vi "HFRR ADV v09.vi"() -> ()   [LabVIEW 2025] (continued)
                }
                n3148 = local read "TITTLE"() -> (w4088:string)
                n3149 = call-dynamic "Set Report Header Text.vi"("report in"=w4071, "center header text"=w4088, "error in (no error)"=w4070) -> ("report out"=w4109:refnum<class "NI_report.lvclass">, "error out"=w4108:errorcluster)  [unwired: 11 in]
                n3150 = for {
                  N: 1 -> [_]
                  tunnel: [w4147] -> w4095
                  tunnel: [w4146] -> w4094
                  tunnel: w4109 -> [w4145]
                  tunnel: w4108 -> [w4144]
                  n3151 = call-dynamic "New Report Line.vi"("report in"=w4145, "error in (no error)"=w4144) -> ("report out"=w4147:refnum<class "NI_report.lvclass">, "error out"=w4146:errorcluster)  [unwired: 12 in]
                }
                n3152 = for {
                  N: 2 -> [_]
                  tunnel: [w4139] -> w4101
                  tunnel: [w4138] -> w4100
                  tunnel: w4095 -> [w4137]
                  tunnel: w4094 -> [w4136]
                  n3153 = call-dynamic "New Report Line.vi"("report in"=w4137, "error in (no error)"=w4136) -> ("report out"=w4139:refnum<class "NI_report.lvclass">, "error out"=w4138:errorcluster)  [unwired: 12 in]
                }
                n3154 = for {
                  N: 25 -> [_]
                  tunnel: w4101 -> [w4135]
                  tunnel: w4100 -> [w4133]
                  tunnel: [w4134] -> w4104
                  tunnel: [w4132] -> w4103
                  n3155 = call-dynamic "Set Report Tab Width.vi"("report in"=w4135, "error in (no error)"=w4133) -> ("report out"=w4134:refnum<class "NI_report.lvclass">, "error out"=w4132:errorcluster)  [unwired: 12 in]
                }
                n3156 = control-ref of="Tab Control 9"() -> (w4099:refnum<vi>)
                n3157 = call-dynamic "Append Control Image to Report.vi"("report in"=w4104, "alignment (default)"=HTML_Report_Image_Alignment."ABSMIDDLE", "ctrl reference"=w4099, "error in (no error)"=w4103) -> ("report out"=w4098:refnum<class "NI_report.lvclass">, "error out"=w4097:errorcluster)  [unwired: 8 in, 2 out]
                n3158 = for {
                  N: 3 -> [_]
                  tunnel: [w4131] -> w4082
                  tunnel: [w4130] -> w4081
                  tunnel: w4098 -> [w4129]
                  tunnel: w4097 -> [w4128]
                  n3159 = call-dynamic "New Report Line.vi"("report in"=w4129, "error in (no error)"=w4128) -> ("report out"=w4131:refnum<class "NI_report.lvclass">, "error out"=w4130:errorcluster)  [unwired: 12 in]
                }
                n3160 = for {
                  N: 100 -> [_]
                  tunnel: w4082 -> [w4127]
                  tunnel: w4081 -> [w4125]
                  tunnel: [w4126] -> w4078
                  tunnel: [w4124] -> w4076
                  n3161 = call-dynamic "Set Report Tab Width.vi"("report in"=w4127, "error in (no error)"=w4125) -> ("report out"=w4126:refnum<class "NI_report.lvclass">, "error out"=w4124:errorcluster)  [unwired: 12 in]
                }
                n3162 = String To Path(string="C:\\LAB-IQ\\im\\Temp_resized.jpg") -> (path=w4068:path)
                n3163 = call-poly <vilib>:"Append Image to Report.vi"("report in"=w4078, "path or URL of image"=w4068, "error in (no error)"=w4076) -> ("report out"=w4077:refnum<class "NI_report.lvclass">, "error out"=w4075:errorcluster)  [unwired: 9 in, 2 out]
                n3164 = call-poly <vilib>:"Open HTML Report in Browser.vi"("report in"=w4077, "error in (no error)"=w4075) -> ("report out"=w4112:refnum<class "NI_report.lvclass">, "error out"=w4111:errorcluster)  [unwired: 11 in, 1 out]
                n3165 = call-dynamic "Dispose Report.vi"("report in"=w4112, "error in (no error)"=w4111) -> ()  [unwired: 13 in, 1 out]
              }
              frame #2 {
              }
              frame #3 {
                n3166 = disable-structure shown="Disabled" {
                  frame Disabled {
                    n3167 = local read "String 10"() -> (w4152:string)
                    n3168 = Concatenate Strings("C:\\LAB-IQ-NXT\\Data\\" ("string"), w4152, ".jpg" ("string")) -> (w4150:string)
                    n3169 = String To Path(string=w4150) -> (path=w4149:path)
                    n3170 = Delete(path (use dialog)=w4149) -> ()  [unwired: 4 in, 3 out]
                  }
                  frame Enabled {
                  }
                }
                n3171 = local write "Print 2"(FALSE ("Print")) -> ()
              }
            }
          }
        }
      }
    }
    n3172 = property on="SetTemp" class="DigNum (strict)"("Disabled"=w2040) -> ()  [unwired: 2 in, 2 out]
    n3173 = Multiply(x=w2029, y=w2031) -> (x*y=w2030:dbl)
    n3174 = local read "MWSD"() -> (w2028:dbl)
    n3175 = Add(x=w2030, y=w2028) -> (x+y=→"WS1.4":dbl)
    n3176 = Wait (ms)(milliseconds to wait=u32 50) -> ()  [unwired: 1 out]
    n3177 = Wait (ms)(milliseconds to wait=u32 50) -> ()  [unwired: 1 out]
    n3178 = local read "Quit"() -> (w2027:bool)
  }
  n3179 = VISA Close(VISA resource name=w48, error in (no error)=w47) -> (error out=w45:errorcluster)
  n3180 = VISA Close(VISA resource name=w29, error in (no error)=w28) -> ()  [unwired: 1 out]
  n3181 = call <vilib>:"Clear Errors.vi"("error in (no error)"=w45) -> ()  [unwired: 5 in, 2 out]
  n3182 = Or(x=w35, y=w34) -> (x .or. y?=w36:bool)
  n3183 = while {
    tunnel: [w4300] -> w41
    shift-right: [w4338] -> _
    shift-left: "" -> [w4326]
    tunnel: [w4314] -> _
    i -> [w4314]
    stop <- w4300 stop-if-true
    w4340 = ";" ("string")
    n3184 = local read "start en"() -> (w4359:bool)
    n3185 = And(x="st enable", y=w4359) -> (x .and. y?=w4360:bool)
    n3186 = local read "ACQUIRE 3"() -> (w4303:bool)
    n3187 = local read "Elapsed time"() -> (w4322:dbl)
    n3188 = case shown="True" w4360 {
      tunnel: "st enable" -> [w4424 w4425]
      tunnel: [w4424 w4425] -> w4304
      frame False {
      }
      frame True {
        n3189 = local write "start en"(FALSE ("start en")) -> ()
      }
    }
    n3190 = Wait (ms)(milliseconds to wait=u32 80) -> ()  [unwired: 1 out]
    n3191 = local read "Stroke"() -> (w4313:dbl)
    n3192 = Greater?(x=w4322, y=0.1) -> (0:w4320:bool)
    n3193 = Or(x=w4304, y=w4303) -> (x .or. y?=w4305:bool)
    n3194 = case shown="True" "ACQUIRE 2" {
      frame False {
      }
      frame True {
        n3195 = call "Elapsed Time13"() -> ("Time has Elapsed"=w4367:bool)  [unwired: 12 in, 7 out]
        n3196 = case shown="True" w4367 {
          frame False {
          }
          frame True {
            n3197 = local write "ACQUIRE 2"(FALSE ("ACQUIRE 2")) -> ()
            n3198 = local write "ACQUIRE 3"(FALSE ("ACQUIRE 2")) -> ()
          }
        }
        n3199 = local write "ACQUIRE 3"(TRUE ("ACQUIRE 2")) -> ()
      }
    }
    n3200 = case shown="True" w4305 {
      tunnel: w4313 -> [_ w4447]
      tunnel: [w4427 _] -> w4357
      tunnel: w4320 -> [_ _]
      tunnel: w4303 -> [_ w4434]
      frame False {
        w4427 = TRUE ("PID Rst")
        n3201 = local read "stop cmd"() -> (w4428:bool)
        n3202 = case shown="True" w4428 {
          frame False {
          }
          frame True {
            n3203 = local write "stop cmd"(FALSE ("stop cmd")) -> ()
          }
        }
        n3204 = local write "PID Rst"(TRUE ("PID Rst")) -> ()
        "start en" <- w4427
      }
      frame True {
        w4454 = cluster{"output high":dbl, "output low":dbl} {"output high"=600.0, "output low"=-600.0} ("output range")
        n3205 = local read "STROKE GAIN :"() -> (w4439:dbl)
        n3206 = call "Elapsed Time6"("Reset"="PID Rst", "Auto Reset"=FALSE) -> ("Time has Elapsed"=w4448:bool)  [unwired: 10 in, 7 out]
        n3207 = Multiply(x="Set Strk", y=w4439) -> (x*y=w4432:dbl)
        n3208 = case shown="False" w4448 {
          tunnel: [w4459 w4460] -> w4451
          tunnel: "Set Strk" -> [w4459 _]
          tunnel: w4447 -> [_ w4460]
          frame False {
          }
          frame True {
          }
        }
        n3209 = Multiply(x=w4432, y=1.0) -> (x*y=w4431:dbl)
        n3210 = Select(t=T8 {"Proportional Gain (Kc)"=0.0, "Integral Time (Ti, min)"=0.02, "Derivative Time (Td, min)"=0.0} ("Stroke PID Gains"), s=w4434, f="Stroke PID Gains") -> (s? t:f=w4435:T8)
        n3211 = Not(x=w4448) -> (.not. x?=w4446:bool)
        n3212 = call-poly <vilib>:"PID.vi"("reinitialize? (F)"=w4446, "output range"=w4454, "PID gains"=w4435, "process variable"=w4451, "setpoint"="Set Strk") -> ("output"=w4445:dbl)  [unwired: 5 in, 1 out]
        "Stroke PID OUT" <- w4445
        n3213 = Select(t=w4445, s=w4448, f=0.0) -> (s? t:f=w4449:dbl)
        n3214 = flat-sequence {
          tunnel: w4449 -> [_]
          frame #0 {
            n3215 = local write "PID Rst"(FALSE ("PID Rst")) -> ()
          }
        }
        n3216 = Add(x=w4431, y=w4449) -> (x+y=w4444:dbl)
        n3217 = Unbundle(w4454) -> ("output high"=w4453:dbl, "output low"=w4452:dbl)
        n3218 = To Word Integer(number=w4444) -> (16bit integer=w4441:i16)
        n3219 = property on="Stroke PID OUT" class="Slide (strict)"("Scale.Range:Minimum"=w4452, "Scale.Range:Maximum"=w4453) -> ()  [unwired: 2 in, 2 out]
        n3220 = In Range and Coerce(upper limit=4095.0 ("f"), x=w4441, lower limit=100.0 ("f")) -> (coerced(x)=w4438:dbl)  [unwired: 1 out]
        "PID Out" <- w4438
        n3221 = Number To Decimal String(number=w4438) -> (decimal integer string=→"st gain":string)  [unwired: 1 in]
        "stop cmd" <- TRUE ("Auto Reset")
      }
    }
    n3222 = flat-sequence {
      frame #0 {
        n3223 = local read "CH-POWER +"() -> (w4371:u16)
        n3224 = local read "CH-POWER -"() -> (w4372:u16)
        n3225 = case shown="1" w4372 {
          tunnel: "PWR" -> [w4373 w4374 w4375 w4376 w4377 w4378 w4379 w4380]
          frame 0, Default {
            n3226 = local write "Do 0"(w4373) -> ()
          }
          frame 1 {
            n3227 = local write "Do 1"(w4374) -> ()
          }
          frame 2 {
            n3228 = local write "Do 2"(w4375) -> ()
          }
          frame 3 {
            n3229 = local write "Do 3"(w4376) -> ()
          }
          frame 4 {
            n3230 = local write "Do 4"(w4377) -> ()
          }
          frame 5 {
            n3231 = local write "Do 5"(w4378) -> ()
          }
          frame 6 {
            n3232 = local write "Do 6"(w4379) -> ()
          }
          frame 7 {
            n3233 = local write "Do 7"(w4380) -> ()
          }
        }
        n3234 = case shown="1" w4371 {
          tunnel: "PWR" -> [w4381 w4382 w4383 w4384 w4385 w4386 w4387 w4388]
          frame 0, Default {
            n3235 = local write "Do 0"(w4381) -> ()
          }
          frame 1 {
            n3236 = local write "Do 1"(w4382) -> ()
          }
          frame 2 {
            n3237 = local write "Do 2"(w4383) -> ()
          }
          frame 3 {
            n3238 = local write "Do 3"(w4384) -> ()
          }
          frame 4 {
            n3239 = local write "Do 4"(w4385) -> ()
          }
          frame 5 {
            n3240 = local write "Do 5"(w4386) -> ()
          }
          frame 6 {
            n3241 = local write "Do 6"(w4387) -> ()
          }
          frame 7 {
            n3242 = local write "Do 7"(w4388) -> ()
          }
        }
      }
    }
    n3243 = local read "RUN"() -> (w4311:bool)
    n3244 = Or(x=w4311, y="ACQUIRE 3") -> (x .or. y?=w4310:bool)
    n3245 = local read "Set Hz"() -> (w4328:dbl)
    n3246 = Select(t=w4328, s=w4310, f=0.0) -> (s? t:f=w4327:dbl)
    n3247 = local read "st gain"() -> (w4331:string)
    n3248 = local read "DO"() -> (w4332:string)
    n3249 = case shown="True" "Boolean 10" {
      frame False {
      }
      frame True {
        n3250 = local write "Tab Control 8"(enum32{"setup", "calibrate"}."calibrate" ("Tab Control 8")) -> ()
        n3251 = local write "Boolean 10"(FALSE ("Boolean 10")) -> ()
      }
    }
    n3252 = Number To Decimal String(number=w4327) -> (decimal integer string=w4330:string)  [unwired: 1 in]
    n3253 = case shown="True" "Boolean 11" {
      frame False {
      }
      frame True {
        n3254 = local write "Tab Control 8"(enum32{"setup", "calibrate"}."setup" ("Tab Control 8")) -> ()
        n3255 = local write "Boolean 11"(FALSE ("Boolean 11")) -> ()
      }
    }
    n3256 = String Length(string=w4331) -> (length=w4346:i32)
    n3257 = String Length(string=w4332) -> (length=w4334:i32)
    n3258 = String Length(string=w4330) -> (length=w4347:i32)
    n3259 = Subtract(x=4.0, y=w4346) -> (x-y=w4343:dbl)
    n3260 = Subtract(x=3.0, y=w4334) -> (x-y=w4337:dbl)
    n3261 = flat-sequence {
      tunnel: w4357 -> [_]
      frame #0 {
        n3262 = Build Array("Do 0", "Do 1", "Do 2", "Do 3", "Do 4", "Do 5", "Do 6", "Do 7") -> (w4415:bool[])
        n3263 = Boolean Array To Number(Boolean array=w4415) -> (number=w4413:u32)
        n3264 = Add(x=w4413, y=u32 0) -> (x+y=w4411:u32)
        n3265 = Number To Decimal String(number=w4411) -> (decimal integer string=→"DO":string)  [unwired: 1 in]
      }
    }
    n3266 = Subtract(x=3.0, y=w4347) -> (x-y=w4348:dbl)
    n3267 = Replace Substring(3:w4343, 4:w4331, 5:"0000" ("string")) -> (1:w4341:string)  [unwired: 1 in, 1 out]
    n3268 = Replace Substring(3:w4337, 4:w4332, 5:"000" ("string")) -> (1:w4333:string)  [unwired: 1 in, 1 out]
    n3269 = Replace Substring(3:w4348, 4:w4330, 5:"000" ("string")) -> (1:w4342:string)  [unwired: 1 in, 1 out]
    n3270 = Concatenate Strings("*" ("string"), w4342, w4340, w4341, w4340, w4333, "$" ("string")) -> (w4338:string)
    "Stroke_send_Val" <- w4338
    n3271 = local read "RUN"() -> (w4308:bool)
    n3272 = local read "ACQUIRE 3"() -> (w4307:bool)
    n3273 = local read "send"() -> (w4324:bool)
    n3274 = Not Equal?(x=w4326, y=w4338) -> (x != y?=w4339:bool)
    n3275 = Or(x=w4308, y=w4307) -> (x .or. y?=w4306:bool)
    n3276 = And(x=w4324, y=w4306) -> (x .and. y?=w4323:bool)
    n3277 = Or(x=w4339, y=w4323) -> (x .or. y?=w4317:bool)
    n3278 = case shown="False" w4306 {
      frame False {
        "send" <- TRUE ("send")
      }
      frame True {
      }
    }
    n3279 = call "Elapsed Time4"("Time Target (s)"=0.5) -> ("Time has Elapsed"=w4315:bool)  [unwired: 11 in, 7 out]
    n3280 = local read "Din"() -> (w4356:u8[])
    n3281 = Or(x=w4315, y=w4317) -> (x .or. y?=w4316:bool)
    n3282 = local read "Quit"() -> (w4300:bool)
    n3283 = Index Array(array=w4356, index=0) -> (element=w4354:u8)
    n3284 = case shown="True" w4316 {
      tunnel: w4338 -> [_ w4392]
      frame False {
      }
      frame True {
        n3285 = local read "Due Com"() -> (w4393:string[])
        n3286 = Build Array (concatenate)(w4393, w4392) -> (→"Due Com":string[])
        n3287 = local write "send"(FALSE ("send")) -> ()
      }
    }
    n3288 = Number To Boolean Array(number=w4354) -> (Boolean array=w4353:bool[])
    n3289 = Array Size(array=w4353) -> (size(s)=w4352:i32)
    n3290 = Greater Than 0?(x=w4352) -> (x > 0?=w4351:bool)
    n3291 = case shown="True" w4351 {
      tunnel: w4353 -> [_ w4407]
      frame False {
      }
      frame True {
        n3292 = Index Array(array=w4407, index #1=0 ("index"), index #2=1 ("index"), index #3=2 ("index"), index #4=3 ("index"), index #5=4 ("index"), index #6=5 ("index"), index #7=6 ("index"), index #8=7 ("index")) -> (element #1=→"DI 0":bool, element #2=→"DI 1":bool, element #3=→"DI 2":bool, element #4=→"DI 3":bool, element #5=→"DI 4":bool, element #6=→"DI 5":bool, element #7=→"DI 6":bool, element #8=→"DI 7":bool)
      }
    }
  }
  n3293 = Or(x=w31, y=w36) -> (x .or. y?=w43:bool)
  n3294 = control-ref of="new picture"() -> ()  [unwired: 1 out]
  n3295 = Or(x=w50, y=w43) -> (x .or. y?=w40:bool)
  n3296 = Or(x=w40, y=w41) -> (x .or. y?=w32:bool)
  n3297 = while {
    tunnel: [w4462] -> w54
    tunnel: [w4463] -> _
    i -> [w4463]
    stop <- w4462 stop-if-true
    n3298 = local read "PID-out"() -> (w4464:dbl)
    "Horizontal Slider Control" <- w4464
    n3299 = Greater Or Equal?(x=w4464, y=2.0) -> (x >= y?=w4465:bool)
    n3300 = flat-sequence {
      tunnel: w4465 -> [w4473]
      tunnel: w4464 -> [w4476]
      tunnel: [w4474] -> w4471
      tunnel: [w4472] -> w4470
      tunnel: [w4492] -> w4469
      tunnel: w4471 -> [w4492]
      tunnel: w4470 -> [w4489]
      tunnel: [w4489] -> w4468
      tunnel: w4469 -> [w4494]
      tunnel: [w4493] -> w4467
      tunnel: w4468 -> [w4493]
      tunnel: w4467 -> [w4508]
      frame #0 {
        n3301 = case shown="True" w4473 {
          selector: w4473 -> [w4478 _]
          frame False {
            n3302 = local write "HEATER"(w4478) -> ()
          }
          frame True {
            w4480 = TRUE ("data")
            n3303 = local read "CH-HEATER"() -> (w4479:u16)
            n3304 = case shown="2" w4479 {
              tunnel: w4480 -> [w4481 w4482 w4483 w4484 w4485 w4486 w4487 w4488]
              frame 0, Default {
                n3305 = local write "Do 0"(w4481) -> ()
              }
              frame 1 {
                n3306 = local write "Do 1"(w4482) -> ()
              }
              frame 2 {
                n3307 = local write "Do 2"(w4483) -> ()
              }
              frame 3 {
                n3308 = local write "Do 3"(w4484) -> ()
              }
              frame 4 {
                n3309 = local write "Do 4"(w4485) -> ()
              }
              frame 5 {
                n3310 = local write "Do 5"(w4486) -> ()
              }
              frame 6 {
                n3311 = local write "Do 6"(w4487) -> ()
              }
              frame 7 {
                n3312 = local write "Do 7"(w4488) -> ()
              }
            }
            "HEATER" <- w4480
          }
        }
        n3313 = Select(t=w4476, s=w4473, f=0.0) -> (s? t:f=w4472:dbl)
        n3314 = Greater Or Equal?(x=w4476, y=97.0) -> (x >= y?=w4474:bool)
      }
      frame #1 {
        n3315 = Multiply(x=w4489, y=5.0) -> (x*y=w4491:dbl)
        n3316 = Wait (ms)(milliseconds to wait=w4491) -> ()  [unwired: 1 out]
      }
      frame #2 {
        n3317 = case shown="False" w4494 {
          frame False {
            w4495 = FALSE ("data")
            n3318 = local read "CH-HEATER"() -> (w4496:u16)
            n3319 = case shown="4" w4496 {
              tunnel: w4495 -> [w4497 w4498 w4499 w4500 w4501 w4502 w4503 w4504]
              frame 0, Default {
                n3320 = local write "Do 0"(w4497) -> ()
              }
              frame 1 {
                n3321 = local write "Do 1"(w4498) -> ()
              }
              frame 2 {
                n3322 = local write "Do 2"(w4499) -> ()
              }
              frame 3 {
                n3323 = local write "Do 3"(w4500) -> ()
              }
              frame 4 {
                n3324 = local write "Do 4"(w4501) -> ()
              }
              frame 5 {
                n3325 = local write "Do 5"(w4502) -> ()
              }
              frame 6 {
                n3326 = local write "Do 6"(w4503) -> ()
              }
              frame 7 {
                n3327 = local write "Do 7"(w4504) -> ()
              }
            }
            n3328 = local write "HEATER"(w4495) -> ()
          }
          frame True {
          }
        }
      }
      frame #3 {
        n3329 = Subtract(x=100, y=w4508) -> (x-y=w4507:dbl)
        n3330 = Multiply(x=w4507, y=5.0) -> (x*y=w4505:dbl)
        n3331 = Wait (ms)(milliseconds to wait=w4505) -> ()  [unwired: 1 out]
      }
    }
    n3332 = local read "Quit"() -> (w4462:bool)
  }
  n3333 = Or(x=w54, y=w32) -> (x .or. y?=w53:bool)
  n3334 = while {
    tunnel: [w4510] -> w49
    i -> [w4517]
    stop <- w4510 stop-if-true
    n3335 = local read "Quit"() -> (w4510:bool)
    n3336 = Equal To 0?(x=w4517) -> (x = 0?=w4515:bool)
    n3337 = call "Elapsed Time3"("Time Target (s)"=45.0, "Auto Reset"=TRUE) -> ("Time has Elapsed"=w4514:bool)  [unwired: 10 in, 7 out]
    n3338 = Wait (ms)(milliseconds to wait=u32 50) -> ()  [unwired: 1 out]
    n3339 = Or(x=w4514, y=w4515) -> (x .or. y?=w4516:bool)
    n3340 = case shown="True" w4516 {
      frame False {
      }
      frame True {
        n3341 = call <vilib>:"System Exec.vi"("run minimized? (F)"=TRUE, "error in (no error)"="error in (no error)", "command line"="powercfg.exe -change -monitor-timeout-ac 0") -> ("error out"=w4528:errorcluster)  [unwired: 5 in, 3 out]
        n3342 = call <vilib>:"System Exec.vi"("run minimized? (F)"=TRUE, "error in (no error)"=w4528, "command line"="powercfg.exe -change -disk-timeout-ac 0") -> ("error out"=w4527:errorcluster)  [unwired: 5 in, 3 out]
        n3343 = call <vilib>:"System Exec.vi"("run minimized? (F)"=TRUE, "error in (no error)"=w4527, "command line"="powercfg.exe -change -standby-timeout-ac 0") -> ("error out"=w4526:errorcluster)  [unwired: 5 in, 3 out]
        n3344 = call <vilib>:"System Exec.vi"("run minimized? (F)"=TRUE, "error in (no error)"=w4526, "command line"="powercfg.exe -change -hibernate-timeout-ac 0") -> ("error out"=w4525:errorcluster)  [unwired: 5 in, 3 out]
        n3345 = call <vilib>:"Simple Error Handler.vi"("error in (no error)"=w4525) -> ("error out"=w4531:errorcluster)  [unwired: 4 in, 4 out]
        n3346 = call <vilib>:"Clear Errors.vi"("error in (no error)"=w4531) -> ("error out"=→"error out":errorcluster)  [unwired: 5 in, 1 out]
      }
    }
  }
  n3347 = Compound Arithmetic op=OR(w52, w53, w49) -> (w51:bool)
  n3348 = flat-sequence {
    tunnel: w51 -> [_]
    tunnel: [w4533] -> w9
    tunnel: w9 -> [_]
    frame #0 {
      n3349 = call "CLOSE CONNECTION.vi"() -> ("error out"=w4533:errorcluster)  [unwired: 11 in]
    }
    frame #1 {
      n3350 = Quit LabVIEW(quit? (T)=TRUE) -> ()
      n3351 = local write "Quit"(FALSE ("EXIT")) -> ()
    }
  }
  n3352 = property on="Heater Button" class="Bool (strict)"("Visible"=TRUE) -> ()  [unwired: 2 in, 2 out]
  n3353 = disable-structure shown="Disabled" {
    disable-tunnel: _ -> [w4539 _]
    disable-tunnel: _ -> [w4536 _]
    disable-tunnel: _ -> [w4537 _]
    frame Disabled {
      n3354 = disable-structure shown="Disabled" {
        disable-tunnel: [w4546 _] -> w4538
        frame Disabled {
          n3355 = while {
            shift-right: [w4588] -> w4544
            shift-left: errorcluster {"status"=TRUE, "code"=0, "source"="Init"} ("error out") -> [w4553]
            shift-right: [w4587] -> w4543
            shift-left: _ -> [w4554]
            shift-right: [w4586] -> _
            shift-left: "" -> [w4585]
            tunnel: [w4547] -> w4546
            shift-right: ["Set Rh"] -> _
            shift-left: 0.0 ("Set Rh") -> [w4579]
            tunnel: [w4556] -> _
            i -> [w4556]
            stop <- w4547 stop-if-true
            n3356 = flat-sequence {
              tunnel: w4553 -> [w4591]
              tunnel: [w4591] -> w4552
              frame #0 {
                n3357 = Wait (ms)(milliseconds to wait=u32 200) -> ()  [unwired: 1 out]
              }
            }
            n3358 = local read "Com Port 3"() -> (w4555:refnum<visa-resource-name>)
            n3359 = local read "Humidity Str Rec"() -> (w4557:string)
            n3360 = Not Equal?(x="Set Rh", y=w4579) -> (x != y?=w4584:bool)
            n3361 = Number To Decimal String(number="Set Rh") -> (decimal integer string=w4582:string)  [unwired: 1 in]
            n3362 = Not Equal?(x=w4555, y=w4554) -> (x != y?=w4550:bool)
            n3363 = Concatenate Strings("#setPoint00" ("string"), w4582) -> (w4583:string)
            n3364 = case shown="False" w4584 {
              tunnel: w4583 -> [_ w4603]
              frame False {
                n3365 = local read "Humidity"() -> (w4600:bool)
                n3366 = case shown="True" w4600 {
                  frame False {
                    n3367 = local write "Humidity Str Send"("stop" ("Humidity Str Send")) -> ()
                  }
                  frame True {
                    n3368 = local write "Humidity Str Send"("start" ("Humidity Str Send")) -> ()
                  }
                }
              }
              frame True {
                n3369 = local write "Humidity Str Send"(w4603) -> ()
              }
            }
            n3370 = Or(x=w4550, y="Re-Initialise") -> (x .or. y?=w4549:bool)
            n3371 = String Subset(string=w4557, offset (0)=7) -> (substring=w4572:string)  [unwired: 1 in]
            n3372 = Match Pattern(string=w4557, regular expression="?") -> (offset past match=w4575:i32)  [unwired: 1 in, 3 out]
            n3373 = Match Pattern(string=w4557, regular expression="v") -> (offset past match=w4578:i32)  [unwired: 1 in, 3 out]
            n3374 = case shown="True" w4549 {
              tunnel: w4552 -> [w4589 _]
              tunnel: [w4589 errorcluster {"status"=TRUE, "code"=0, "source"="Init"} ("error out")] -> w4551
              frame False {
              }
              frame True {
              }
            }
            n3375 = Equal?(x=w4575, y=-1) -> (x = y?=w4559:bool)
            n3376 = Match Pattern(string=w4572, regular expression="g") -> (after substring=w4573:string, offset past match=w4564:i32)  [unwired: 1 in, 2 out]
            n3377 = Match Pattern(string=w4572, regular expression="y") -> (after substring=w4571:string, offset past match=w4565:i32)  [unwired: 1 in, 2 out]
            n3378 = Greater?(x=w4565, y=w4564) -> (0:w4570:bool)
            n3379 = Greater Or Equal To 0?(x=w4565) -> (x >= 0?=w4562:bool)
            n3380 = Greater Or Equal To 0?(x=w4564) -> (x >= 0?=w4563:bool)
            n3381 = Or(x=w4562, y=w4563) -> (x .or. y?=w4561:bool)
            n3382 = Greater Or Equal To 0?(x=w4578) -> (x >= 0?=w4560:bool)
            n3383 = Select(t=w4571, s=w4570, f=w4573) -> (s? t:f=w4566:string)
            n3384 = case shown="Error" w4551 {
              selector: w4551 -> [w4616 w4662]
              tunnel: [w4614 w4655] -> w4588
              tunnel: w4554 -> [w4617 w4661]
              tunnel: [w4615 w4664] -> w4587
              tunnel: w4585 -> [w4604 w4663]
              tunnel: [w4611 w4663] -> w4586
              frame No Error {
                n3385 = call "Elapsed Time7"() -> ("Time has Elapsed"=w4610:bool)  [unwired: 12 in, 7 out]
                n3386 = Not Equal?(x="Humidity Str Send", y=w4604) -> (x != y?=w4606:bool)
                n3387 = Or(x=w4606, y=w4610) -> (x .or. y?=w4609:bool)
                n3388 = Select(t="Humidity Str Send", s=w4606, f="vals" ("regular expression")) -> (s? t:f=w4605:string)
                n3389 = Or(x=w4609, y="Send") -> (x .or. y?=w4613:bool)
                n3390 = case shown="True" w4613 {
                  tunnel: [w4620 w4625] -> w4614
                  tunnel: w4617 -> [w4619 w4633]
                  tunnel: w4616 -> [w4620 w4632]
                  tunnel: [w4619 w4626] -> w4615
                  tunnel: w4605 -> [_ w4631]
                  tunnel: [w4618 w4622] -> w4611
                  tunnel: "Humidity Str Send" -> [_ w4623]
                  tunnel: w4606 -> [_ w4624]
                  tunnel: w4604 -> [w4618 w4621]
                  frame False {
                  }
                  frame True {
                    n3391 = flat-sequence {
                      tunnel: w4633 -> [w4641]
                      tunnel: w4632 -> [w4640]
                      tunnel: w4631 -> [w4637]
                      tunnel: [w4639] -> w4630
                      tunnel: [w4638] -> w4629
                      tunnel: w4630 -> [w4644]
                      tunnel: w4629 -> [w4643]
                      tunnel: [w4644] -> w4628
                      tunnel: [w4643] -> w4627
                      tunnel: w4628 -> [w4651]
                      tunnel: w4627 -> [w4650]
                      tunnel: [w4649] -> w4626
                      tunnel: [w4648] -> w4625
                      frame #0 {
                        n3392 = local write "Ser Led"(TRUE ("Boolean 4")) -> ()
                        n3393 = Concatenate Strings(w4637, "\r") -> (w4636:string)
                        n3394 = VISA Write(VISA resource name=w4641, write buffer=w4636, error in (no error)=w4640) -> (VISA resource name out=w4639:refnum<visa-resource-name>, error out=w4638:errorcluster)  [unwired: 1 out]
                      }
                      frame #1 {
                        n3395 = Wait (ms)(milliseconds to wait="wait") -> ()  [unwired: 1 out]
                      }
                      frame #2 {
                        w4646 = FALSE ("Send")
                        n3396 = property class="Instr"(reference=w4651, error in=w4650) -> (reference out=w4652:refnum<visa-resource-name>, error out=w4653:errorcluster, "Serial Settings:Number of Bytes at Serial Port"=w4645:u32)
                        "Humidity 2" <- w4645
                        n3397 = local write "Send"(w4646) -> ()
                        n3398 = local write "Ser Led"(w4646) -> ()
                        n3399 = VISA Read(VISA resource name=w4652, byte count=w4645, error in (no error)=w4653) -> (VISA resource name out=w4649:refnum<visa-resource-name>, read buffer=→"Humidity Str Rec":string, error out=w4648:errorcluster)  [unwired: 1 out]
                      }
                    }
                    n3400 = Select(t=w4623, s=w4624, f=w4621) -> (s? t:f=w4622:string)
                  }
                }
              }
              frame Error {
                w4669 = u16 0 items=["None"=0, "XON/XOFF"=1, "RTS/CTS"=2, "DTR/DSR"=4] ("flow control")
                w4665 = u16 0 items=["None", "Odd", "Even", "Mark", "Space"] ("parity")
                w4668 = u16 10 items=["1.0"=10, "1.5"=15, "2.0"=20] ("stop bits")
                n3401 = VISA Close(VISA resource name=w4661, error in (no error)=w4662) -> (error out=w4660:errorcluster)
                n3402 = local write "humid"("" ("humid")) -> ()
                n3403 = local write "Humidity Str Rec"("" ("Humidity Str Rec")) -> ()
                n3404 = call <vilib>:"Clear Errors.vi"("error in (no error)"=w4660) -> ("error out"=w4659:errorcluster)  [unwired: 5 in, 1 out]
                n3405 = local read "Com Port 3"() -> (w4658:refnum<visa-resource-name>)
                n3406 = call-poly "VISA Configure Serial Port"("VISA resource name"=w4658, "timeout (10sec)"=u32 1000, "termination char\n(0xA = '\\n' = LF)"=u8 10 ("termination char\n(0xA = '\\n' = LF)"), "Enable Termination\nChar (T)"=FALSE ("Enable Termination Char (T)"), "baud rate (9600)"="Humidity BaudRate", "data bits (8)"=u16 8 ("data bits"), "parity (0:none)"=w4665, "error in (no error)"=w4659, "stop bits (10: 1 bit)"=w4668, "flow control (0:none)"=w4669) -> ("VISA resource name out"=w4664:refnum<visa-resource-name>, "error out"=w4655:errorcluster)  [unwired: 4 in]
              }
            }
            n3407 = Compound Arithmetic op=AND(w4560, w4559, w4561) -> (w4558:bool)
            n3408 = case shown="True" w4558 {
              tunnel: w4557 -> [_ _]
              tunnel: w4566 -> [_ w4596]
              frame False {
              }
              frame True {
                w4594 = " " ("regular expression")
                n3409 = Match Pattern(string=w4596, regular expression=" ") -> (after substring=w4598:string)  [unwired: 1 in, 3 out]
                n3410 = Match Pattern(string=w4598, regular expression=w4594) -> (before substring=→"humid":string, after substring=w4595:string)  [unwired: 1 in, 2 out]
                n3411 = Match Pattern(string=w4595, regular expression=w4594) -> (before substring=→"temp_@Rh sensor":string)  [unwired: 1 in, 3 out]
              }
            }
            n3412 = local read "Quit"() -> (w4547:bool)
          }
          n3413 = VISA Close(VISA resource name=w4543, error in (no error)=w4544) -> (error out=w4540:errorcluster)
          n3414 = call <vilib>:"Clear Errors.vi"("error in (no error)"=w4540) -> ()  [unwired: 5 in, 2 out]
        }
        frame Enabled {
        }
      }
    }
    frame Enabled {
    }
  }
  n3415 = while {
    tunnel: [w4677] -> _
    i -> [w4677]
    stop <- w4672 stop-if-true
    # "Langauage selection"
    n3416 = property on="FF Calibration g" class="WFGraph (strict)"("Plot Area:Colors:FG Color"=u32 0) -> ()  [unwired: 2 in, 2 out]
    n3417 = Equal?(x="Lan flag", y=22.0) -> ()  [unwired: 1 out]
    n3418 = disable-structure shown="Disabled" {
      frame Disabled {
        n3419 = stacked-sequence {
          frame #0 {
            n3420 = case shown="\"Russian\"" "Language Selection" {
              tunnel: [0 1] -> w4679
              frame "English", Default {
              }
              frame "Russian" {
              }
            }
            n3421 = for {
              N: 130 -> [_]
              tunnel: "Table" -> [w4688]
              tunnel: w4679 -> [w4687]
              i -> [w4686]
              n3422 = Index Array(array=w4688, index (row)=w4686, index (col)=w4687) -> (element=w4685:string)
              n3423 = case shown="4" w4686 {
                tunnel: w4685 -> [w4689 w4690 _ w4691 w4692 w4693 w4694 w4695 w4696 w4697 w4698 w4699 w4700 w4701 w4702 w4703 w4704 w4705 w4706 w4707 w4708 w4709 w4710 w4711 w4712 w4713 w4714 w4715 w4716 _ _ w4717 w4718 w4719 w4720 w4721 w4722 w4731 w4738 w4745 w4752 w4756 w4759 w4762 w4764 w4766 w4767 w4768 w4769 w4770 w4771 w4772 w4773 w4774 w4775 w4776 w4777 w4778 w4779 w4780 w4781 w4782 w4783 w4784 w4785 w4786 w4787 w4788 w4789 w4790 w4791 w4792 w4793 w4794 w4795 w4796 w4797 w4798 w4799 w4800 w4801 w4802 w4803 w4804 w4805 w4806 w4807 w4808 w4809 w4810 w4811 w4812 w4813 w4814 w4815 w4816 w4817 w4818 w4819 w4820 w4821 w4822 w4823 w4824 w4825 _ w4826 w4827 w4828 w4829 w4830 w4831 w4832 w4833 w4834 w4835 w4836 w4837 w4838 _ w4839 w4840 w4841 w4842 w4843 w4844 _]
                frame 0 {
                  n3424 = local write "S"(w4689) -> ()
                }
                frame 1 {
                  n3425 = local write "S 2"(w4690) -> ()
                }
                frame 2 {
                }
                frame 3 {
                  n3426 = local write "S 4"(w4691) -> ()
                }
                frame 4 {
                  n3427 = property on="FILE" class="Str"("Caption.Text"=w4692) -> ()  [unwired: 2 in, 2 out]
                }
                frame 5 {
                  n3428 = property on="Fuel Discription :" class="Str"("Caption.Text"=w4693) -> ()  [unwired: 2 in, 2 out]
                }
                frame 6 {
                  n3429 = property on="Remarks :" class="Str"("Caption.Text"=w4694) -> ()  [unwired: 2 in, 2 out]
                }
                frame 7 {
                  n3430 = property on="Save & Continue" class="Bool (strict)"("Boolean Text.Text"=w4695) -> ()  [unwired: 2 in, 2 out]
                }
                frame 8 {
                }
                frame 9 {
                  n3431 = property on="Set Hz" class="DigNum (strict)"("Caption.Text"=w4697) -> ()  [unwired: 2 in, 2 out]
                }
                frame 10 {
                  "String 3" <- w4698
                }
                frame 11 {
                  n3432 = property on="NORMAL LOAD" class="DigNum (strict)"("Caption.Text"=w4699) -> ()  [unwired: 2 in, 2 out]
                }
                frame 12 {
                  "String 5" <- w4700
                }
                frame 13 {
                  n3433 = property on="Set Temp" class="DigNum (strict)"("Caption.Text"=w4701) -> ()  [unwired: 2 in, 2 out]
                }
                frame 14 {
                  n3434 = local write "S 15"(w4702) -> ()
                }
                frame 15 {
                  n3435 = property on="Set Rh" class="DigNum (strict)"("Caption.Text"=w4703) -> ()  [unwired: 2 in, 2 out]
                }
                frame 16 {
                  "String 13" <- w4704
                  "String 26" <- w4704
                }
                frame 17 {
                  n3436 = local write "S 18"(w4705) -> ()
                }
                frame 18 {
                  "String 17" <- w4706
                }
                frame 19 {
                  n3437 = property on="test time" class="DigNum (strict)"("Caption.Text"=w4707) -> ()  [unwired: 2 in, 2 out]
                }
                frame 20 {
                  "String 18" <- w4708
                  "String 22" <- w4708
                }
                frame 21 {
                  n3438 = property on="Elapsed time" class="DigNum (strict)"("Caption.Text"=w4709) -> ()  [unwired: 2 in, 2 out]
                }
                frame 22 {
                  n3439 = property on="Samplingtime 2" class="DigNum (strict)"("Caption.Text"=w4710) -> ()  [unwired: 2 in, 2 out]
                }
                frame 23 {
                  "String 21" <- w4711
                }
                frame 24 {
                  n3440 = property on="Countdown" class="DigNum (strict)"("Caption.Text"=w4712) -> ()  [unwired: 2 in, 2 out]
                }
                frame 25 {
                  n3441 = property on="Countdown 2" class="DigNum (strict)"("Caption.Text"=w4713) -> ()  [unwired: 2 in, 2 out]
                }
                frame 26 {
                  n3442 = property on="Engage" class="Bool (strict)"("Boolean Text.Text"=w4714) -> ()  [unwired: 2 in, 2 out]
                }
                frame 27 {
                  n3443 = property on="Boolean  4" class="Bool (strict)"("Boolean Text.Text"=w4715) -> ()  [unwired: 2 in, 2 out]
                }
                frame 28 {
                  n3444 = property on="Test \nStatus" class="Bool (strict)"("Boolean Text.Text"=w4716) -> ()  [unwired: 2 in, 2 out]
                }
                frame 29 {
                }
                frame 30 {
                }
                frame 31 {
                  n3445 = property on="FF Calibration g" class="WFGraph (strict)"("X Scale.Name Label.Text"=w4717) -> ()  [unwired: 2 in, 2 out]
                }
                frame 32 {
                  n3446 = property on="RSTCOF" class="Bool"("Boolean Text.Text"=w4718) -> ()  [unwired: 2 in, 2 out]
                  n3447 = property on="RST FF" class="Bool"("Boolean Text.Text"=w4718) -> ()  [unwired: 2 in, 2 out]
                  n3448 = property on="RST TEMP" class="Bool"("Boolean Text.Text"=w4718) -> ()  [unwired: 2 in, 2 out]
                  n3449 = property on="RSTV1 3" class="Bool"("Boolean Text.Text"=w4718) -> ()  [unwired: 2 in, 2 out]
                  n3450 = property on="rstv2" class="Bool"("Boolean Text.Text"=w4718) -> ()  [unwired: 2 in, 2 out]
                  n3451 = property on="RSTV1 2" class="Bool"("Boolean Text.Text"=w4718) -> ()  [unwired: 2 in, 2 out]
                  n3452 = property on="RST CP" class="Bool"("Boolean Text.Text"=w4718) -> ()  [unwired: 2 in, 2 out]
                }
                frame 33 {
                  "S 61" <- w4719
                }
                frame 34 {
                  "String 23" <- w4720
                }
                frame 35 {
                  n3453 = property on="Rh Before" class="DigNum (strict)"("Caption.Text"=w4721) -> ()  [unwired: 2 in, 2 out]
                }
                frame 36 {
                  n3454 = Match Pattern(string=w4722, regular expression=",") -> (before substring=→"bs":string, after substring=→"as":string)  [unwired: 1 in, 2 out]
                  n3455 = property on="Rh After" class="DigNum (strict)"("Caption.Text"=w4722) -> ()  [unwired: 2 in, 2 out]
                }
                frame 37 {
                  n3456 = Match Pattern(string=w4731, regular expression=",") -> (before substring=w4730:string, after substring=w4729:string)  [unwired: 1 in, 2 out]
                  "bs" <- w4730
                  "as" <- w4729
                  n3457 = Concatenate Strings(w4730, w4729) -> (w4726:string)
                  n3458 = property on="Humidity before test 2" class="DigNum (strict)"("Caption.Text"=w4726) -> ()  [unwired: 2 in, 2 out]
                  n3459 = property on="Humidity before test" class="DigNum (strict)"("Caption.Text"=w4726) -> ()  [unwired: 2 in, 2 out]
                  n3460 = Concatenate Strings(w4726, "=" ("string")) -> (w4727:string)
                  n3461 = local write "S 38"(w4727) -> ()
                }
                frame 38 {
                  n3462 = Match Pattern(string=w4738, regular expression=",") -> (before substring=w4737:string, after substring=w4736:string)  [unwired: 1 in, 2 out]
                  "bs" <- w4737
                  "as" <- w4736
                  n3463 = Concatenate Strings(w4737, w4736) -> (w4733:string)
                  n3464 = property on="Humidity after test 2" class="DigNum (strict)"("Caption.Text"=w4733) -> ()  [unwired: 2 in, 2 out]
                  n3465 = Concatenate Strings(w4733, "=" ("string")) -> (w4735:string)
                  n3466 = property on="Humidity after test" class="DigNum (strict)"("Caption.Text"=w4733) -> ()  [unwired: 2 in, 2 out]
                  n3467 = local write "S 39"(w4735) -> ()
                }
                frame 39 {
                  n3468 = Match Pattern(string=w4745, regular expression=",") -> (before substring=w4744:string, after substring=w4743:string)  [unwired: 1 in, 2 out]
                  "bs" <- w4744
                  "as" <- w4743
                  n3469 = Concatenate Strings(w4744, w4743) -> (w4740:string)
                  n3470 = property on="Temperature before test 2" class="DigNum (strict)"("Caption.Text"=w4740) -> ()  [unwired: 2 in, 2 out]
                  n3471 = property on="Temperature before test" class="DigNum (strict)"("Caption.Text"=w4740) -> ()  [unwired: 2 in, 2 out]
                  n3472 = Concatenate Strings(w4740, "=" ("string")) -> (→"String 34":string)
                }
                frame 40 {
                  n3473 = Match Pattern(string=w4752, regular expression=",") -> (before substring=w4751:string, after substring=w4750:string)  [unwired: 1 in, 2 out]
                  "bs" <- w4751
                  "as" <- w4750
                  n3474 = Concatenate Strings(w4751, w4750) -> (w4747:string)
                  n3475 = property on="Temperature after test 2" class="DigNum (strict)"("Caption.Text"=w4747) -> ()  [unwired: 2 in, 2 out]
                  n3476 = Concatenate Strings(w4747, "=" ("string")) -> (→"String 35":string)
                  n3477 = property on="Temperature after test" class="DigNum (strict)"("Caption.Text"=w4747) -> ()  [unwired: 2 in, 2 out]
                }
                frame 41 {
                  n3478 = property on="AVP" class="DigNum (strict)"("Caption.Text"=w4756) -> ()  [unwired: 2 in, 2 out]
                  n3479 = property on="AVP 2" class="DigNum (strict)"("Caption.Text"=w4756) -> ()  [unwired: 2 in, 2 out]
                  n3480 = Concatenate Strings(w4756, "=" ("string")) -> (→"String 36":string)
                }
                frame 42 {
                  n3481 = property on="MWSD" class="DigNum (strict)"("Caption.Text"=w4759) -> ()  [unwired: 2 in, 2 out]
                  n3482 = property on="MWSD 2" class="DigNum (strict)"("Caption.Text"=w4759) -> ()  [unwired: 2 in, 2 out]
                  n3483 = Concatenate Strings(w4759, "=" ("string")) -> (→"String 37":string)
                }
                frame 43 {
                  n3484 = property on="HCF 2" class="DigNum (strict)"("Caption.Text"=w4762) -> ()  [unwired: 2 in, 2 out]
                  n3485 = property on="HCF" class="DigNum (strict)"("Caption.Text"=w4762) -> ()  [unwired: 2 in, 2 out]
                  n3486 = Concatenate Strings(w4762, "=" ("string")) -> (→"String 38":string)
                }
                frame 44 {
                  n3487 = Concatenate Strings(w4764, "=" ("string")) -> (→"String 39":string)
                  n3488 = property on="WS1.4 2" class="DigNum (strict)"("Caption.Text"=w4764) -> ()  [unwired: 2 in, 2 out]
                  n3489 = property on="WS1.4" class="DigNum (strict)"("Caption.Text"=w4764) -> ()  [unwired: 2 in, 2 out]
                }
                frame 45 {
                  n3490 = property on="Save Results" class="Bool (strict)"("Boolean Text.Text"=w4766) -> ()  [unwired: 2 in, 2 out]
                }
                frame 46 {
                  n3491 = local write "S 47"(w4767) -> ()
                }
                frame 47 {
                  n3492 = local write "S 48"(w4768) -> ()
                }
                frame 48 {
                  n3493 = local write "S 49"(w4769) -> ()
                }
                frame 49 {
                  n3494 = local write "S 50"(w4770) -> ()
                }
                frame 50 {
                  n3495 = local write "S 51"(w4771) -> ()
                }
                frame 51 {
                  n3496 = local write "S 52"(w4772) -> ()
                }
                frame 52 {
                  n3497 = local write "S 53"(w4773) -> ()
                }
                frame 53 {
                  n3498 = local write "S 54"(w4774) -> ()
                }
                frame 54 {
                  n3499 = local write "S 55"(w4775) -> ()
                }
                frame 55 {
                  n3500 = local write "S 56"(w4776) -> ()
                }
                frame 56 {
                  n3501 = local write "S 57"(w4777) -> ()
                }
                frame 57 {
                  n3502 = local write "S 58"(w4778) -> ()
                }
                frame 58 {
                  n3503 = local write "S 59"(w4779) -> ()
                }
                frame 59 {
                  n3504 = local write "S 60"(w4780) -> ()
                }
                frame 60 {
                  n3505 = local write "S 62"(w4781) -> ()
                }
                frame 61 {
                  n3506 = local write "S 63"(w4782) -> ()
                }
                frame 62 {
                  n3507 = local write "S 64"(w4783) -> ()
                }
                frame 63 {
                  n3508 = local write "S 65"(w4784) -> ()
                }
                frame 64 {
                  n3509 = local write "S 66"(w4785) -> ()
                }
                frame 65 {
                  n3510 = local write "S 67"(w4786) -> ()
                }
                frame 66 {
                  n3511 = local write "S 68"(w4787) -> ()
                }
                frame 67 {
                  n3512 = local write "S 69"(w4788) -> ()
                }
                frame 68 {
                  n3513 = local write "S 70"(w4789) -> ()
                }
                frame 69 {
                  n3514 = local write "S 71"(w4790) -> ()
                }
                frame 70 {
                  n3515 = local write "S 72"(w4791) -> ()
                }
                frame 71 {
                  n3516 = local write "S 73"(w4792) -> ()
                }
                frame 72 {
                  n3517 = local write "S 74"(w4793) -> ()
                }
                frame 73 {
                  n3518 = local write "S 75"(w4794) -> ()
                }
                frame 74 {
                  n3519 = local write "S 76"(w4795) -> ()
                }
                frame 75 {
                  n3520 = local write "S 77"(w4796) -> ()
                }
                frame 76 {
                  n3521 = local write "S 78"(w4797) -> ()
                }
                frame 77 {
                  n3522 = local write "S 79"(w4798) -> ()
                }
                frame 79 {
                  n3523 = property on="Sample Temperature ( °C )" class="XYGraph (strict)"("Y Scale.Name Label.Text"=w4799) -> ()  [unwired: 2 in, 2 out]
                }
                frame 80 {
                  n3524 = local write "S 81"(w4800) -> ()
                  n3525 = property on="Humidity ( %RH )" class="XYGraph (strict)"("Y Scale.Name Label.Text"=w4800) -> ()  [unwired: 2 in, 2 out]
                }
                frame 78 {
                  n3526 = property on="Air Temperature  ( °C )" class="XYGraph (strict)"("X Scale.Name Label.Text"=w4801) -> ()  [unwired: 2 in, 2 out]
                  n3527 = property on="Humidity ( %RH )" class="XYGraph (strict)"("X Scale.Name Label.Text"=w4801) -> ()  [unwired: 2 in, 2 out]
                  n3528 = property on="Sample Temperature ( °C )" class="XYGraph (strict)"("X Scale.Name Label.Text"=w4801) -> ()  [unwired: 2 in, 2 out]
                  n3529 = property on="Coefficient Of Friction" class="XYGraph (strict)"("X Scale.Name Label.Text"=w4801) -> ()  [unwired: 2 in, 2 out]
                }
                frame 81 {
                  n3530 = property on="Air Temperature  ( °C )" class="XYGraph (strict)"("Y Scale.Name Label.Text"=w4802) -> ()  [unwired: 2 in, 2 out]
                }
                frame 82 {
                  n3531 = local write "S 84"(w4803) -> ()
                }
                frame 83 {
                  n3532 = local write "S 85"(w4804) -> ()
                }
                frame 84 {
                  n3533 = local write "S 86"(w4805) -> ()
                }
                frame 85 {
                  n3534 = local write "S 87"(w4806) -> ()
                }
                frame 86 {
                  n3535 = local write "S 88"(w4807) -> ()
                }
                frame 87 {
                  n3536 = property on="FF Calibration g" class="WFGraph (strict)"("Y Scale.Name Label.Text"=w4808) -> ()  [unwired: 2 in, 2 out]
                }
                frame 88 {
                  n3537 = local write "S 90"(w4809) -> ()
                }
                frame 89 {
                  n3538 = local write "S 91"(w4810) -> ()
                }
                frame 90 {
                  n3539 = local write "S 92"(w4811) -> ()
                }
                frame 91 {
                  n3540 = local write "S 93"(w4812) -> ()
                }
                frame 92 {
                  n3541 = local write "S 94"(w4813) -> ()
                }
                frame 93 {
                  n3542 = local write "S 95"(w4814) -> ()
                }
                frame 94 {
                  n3543 = local write "S 96"(w4815) -> ()
                }
                frame 95 {
                  n3544 = local write "S 97"(w4816) -> ()
                }
                frame 96 {
                  n3545 = local write "S 98"(w4817) -> ()
                }
                frame 97 {
                  n3546 = local write "S 99"(w4818) -> ()
                }
                frame 98 {
                  n3547 = local write "S 100"(w4819) -> ()
                }
                frame 99 {
                  n3548 = local write "S 101"(w4820) -> ()
                }
                frame 100 {
                  n3549 = local write "S 102"(w4821) -> ()
                }
                frame 101 {
                  n3550 = local write "S 103"(w4822) -> ()
                }
                frame 102 {
                  n3551 = local write "S 104"(w4823) -> ()
                }
                frame 103 {
                  n3552 = local write "S 105"(w4824) -> ()
                }
                frame 104 {
                  n3553 = local write "S 106"(w4825) -> ()
                }
                frame 105 {
                }
                frame 106 {
                  n3554 = property on="OK Button 17" class="Bool (strict)"("Boolean Text.Text"=w4826) -> ()  [unwired: 2 in, 2 out]
                }
                frame 107 {
                  n3555 = property on="OK Button 16" class="Bool (strict)"("Boolean Text.Text"=w4827) -> ()  [unwired: 2 in, 2 out]
                }
                frame 108 {
                  n3556 = property on="TITTLE" class="Str"("Caption.Text"=w4828) -> ()  [unwired: 2 in, 2 out]
                }
                frame 109 {
                  "String 30" <- w4829
                }
                frame 110 {
                  n3557 = property on="Test Date" class="Str"("Caption.Text"=w4830) -> ()  [unwired: 2 in, 2 out]
                  "String 31" <- w4830
                }
                frame 111 {
                  n3558 = property on="Sample ID" class="Str"("Caption.Text"=w4831) -> ()  [unwired: 2 in, 2 out]
                  "String 32" <- w4831
                }
                frame 112 {
                  n3559 = property on="Tested by" class="Str"("Caption.Text"=w4832) -> ()  [unwired: 2 in, 2 out]
                  "String 33" <- w4832
                }
                frame 113 {
                  n3560 = property on="System Configured Printers 2" class="Arr (strict)"("Caption.Text"=w4833) -> ()  [unwired: 2 in, 2 out]
                }
                frame 114 {
                  n3561 = property on="Selected Printer" class="Str"("Caption.Text"=w4834) -> ()  [unwired: 2 in, 2 out]
                }
                frame 115 {
                  n3562 = property on="Select Printer 3" class="DigNum (strict)"("Caption.Text"=w4835) -> ()  [unwired: 2 in, 2 out]
                }
                frame 116 {
                  n3563 = property on="Print" class="Bool (strict)"("Boolean Text.Text"=w4836) -> ()  [unwired: 2 in, 2 out]
                }
                frame 117 {
                  "String 41" <- w4837
                }
                frame 118 {
                  n3564 = property on="tested by" class="Str"("Caption.Text"=w4838) -> ()  [unwired: 2 in, 2 out]
                }
                frame 119 {
                }
                frame 120 {
                  n3565 = property on="Export" class="Bool (strict)"("Boolean Text.Text"=w4839) -> ()  [unwired: 2 in, 2 out]
                }
                frame 121 {
                  n3566 = property on="TEMP INTERCEPT:" class="DigNum (strict)"("Caption.Text"=w4840) -> ()  [unwired: 2 in, 2 out]
                }
                frame 122 {
                  n3567 = property on="AIR TEMP INTERCEPT:" class="DigNum (strict)"("Caption.Text"=w4841) -> ()  [unwired: 2 in, 2 out]
                }
                frame 123 {
                  n3568 = property on="Select File Type" class="Enum (strict)"("Caption.Text"=w4842) -> ()  [unwired: 2 in, 2 out]
                }
                frame 124 {
                  n3569 = property on="s.NO" class="Str"("Caption.Text"=w4843) -> ()  [unwired: 2 in, 2 out]
                  "String 45" <- w4843
                }
                frame 125 {
                  n3570 = property on="trip1 8" class="Bool (strict)"("Boolean Text.Text"=w4844) -> ()  [unwired: 2 in, 2 out]
                }
                frame 126, Default {
                }
              }
            }
          }
          frame #1 {
            w4852 = TRUE ("Visible")
            n3571 = local read "S 91"() -> (w4869:string)
            n3572 = local read "S 90"() -> (w4868:string)
            n3573 = local read "S 88"() -> (w4867:string)
            n3574 = property on="Threshold" class="DigNum (strict)"("Caption.Text"=w4869) -> ()  [unwired: 2 in, 2 out]
            n3575 = property on="File Path" class="Path"("Caption.Text"=w4868) -> ()  [unwired: 2 in, 2 out]
            n3576 = property on="SrvM CP" class="Bool (strict)"("Boolean Text.Text"=w4867) -> ()  [unwired: 2 in, 2 out]
            n3577 = local read "S 71"() -> (w4862:string)
            n3578 = local read "S 86"() -> (w4864:string)
            n3579 = local read "S 85"() -> (w4865:string)
            n3580 = local read "S 87"() -> (w4863:string)
            n3581 = local read "S 84"() -> (w4866:string)
            n3582 = local read "S 103"() -> (w4851:string)
            n3583 = local read "S 104"() -> (w4850:string)
            n3584 = property on="ENTER THE NEW PASSWORD" class="Str"("Caption.Text"=w4863) -> ()  [unwired: 2 in, 2 out]
            n3585 = property on="Password" class="Str"("Caption.Text"=w4865) -> ()  [unwired: 2 in, 2 out]
            n3586 = property on="ENTER CURRENT PASSWORD" class="Str"("Caption.Text"=w4864) -> ()  [unwired: 2 in, 2 out]
            n3587 = property on="EDIT" class="Bool (strict)"("Boolean Text.Text"=w4862) -> ()  [unwired: 2 in, 2 out]
            n3588 = property on="SAVE" class="Bool (strict)"("Boolean Text.Text"=w4866) -> ()  [unwired: 2 in, 2 out]
            n3589 = Build Array(w4851, w4850) -> (w4849:string[])
            n3590 = property on="Heater Button" class="Bool (strict)"("Strings [4]"=w4849) -> ()  [unwired: 2 in, 2 out]
            n3591 = property on="CH-HUMIDITY WET" class="DigNum (strict)"("Caption.Size to Text?"=w4852) -> ()  [unwired: 2 in, 2 out]
            n3592 = property on="CH-HUMIDITY DRY" class="DigNum (strict)"("Caption.Size to Text?"=w4852) -> ()  [unwired: 2 in, 2 out]
            n3593 = property on="CH-POWER -" class="DigNum (strict)"("Caption.Size to Text?"=w4852) -> ()  [unwired: 2 in, 2 out]
            n3594 = property on="CH-HEATER" class="DigNum (strict)"("Caption.Size to Text?"=w4852) -> ()  [unwired: 2 in, 2 out]
            n3595 = property on="CH-POWER +" class="DigNum (strict)"("Caption.Size to Text?"=w4852) -> ()  [unwired: 2 in, 2 out]
            n3596 = local read "S 92"() -> (w4861:string)
            n3597 = local read "S 93"() -> (w4860:string)
            n3598 = local read "S 105"() -> (w4847:string)
            n3599 = local read "S 106"() -> (w4846:string)
            n3600 = Build Array(w4861, w4860) -> ()  [unwired: 1 out]
            n3601 = Build Array(w4847, w4846) -> (w4848:string[])
            n3602 = local read "S 95"() -> (w4858:string)
            n3603 = local read "S 94"() -> (w4859:string)
            n3604 = local read "bs"() -> (w4874:string)
            n3605 = local read "as"() -> (w4875:string)
            n3606 = property on="Humidity" class="Bool (strict)"("Strings [4]"=w4848) -> ()  [unwired: 2 in, 2 out]
            n3607 = Concatenate Strings(w4874, "\r", w4875) -> ()  [unwired: 1 out]
            n3608 = property on="STROKE GAIN :" class="DigNum (strict)"("Caption.Text"=w4858) -> ()  [unwired: 2 in, 2 out]
            n3609 = property on="DISPLACEMENT :" class="DigNum (strict)"("Caption.Text"=w4859) -> ()  [unwired: 2 in, 2 out]
            n3610 = property on="Rh After" class="DigNum (strict)"("Caption.Size to Text?"=TRUE ("Caption.Size to Text")) -> ()  [unwired: 2 in, 2 out]
            n3611 = local read "S 48"() -> (w4898:string)
            n3612 = local read "S 50"() -> (w4896:string)
            n3613 = local read "S 51"() -> (w4895:string)
            n3614 = local read "S 49"() -> (w4897:string)
            n3615 = local read "S 52"() -> (w4894:string)
            n3616 = local read "as"() -> (w4879:string)
            n3617 = local read "bs"() -> (w4880:string)
            n3618 = local read "S 56"() -> (w4893:string)
            n3619 = local read "S 57"() -> (w4892:string)
            n3620 = local read "S 58"() -> (w4891:string)
            n3621 = local read "S 59"() -> (w4890:string)
            n3622 = property on="OPEN" class="Bool (strict)"("Boolean Text.Text"=w4894) -> ()  [unwired: 2 in, 2 out]
            n3623 = property on="OPEN 1" class="Bool (strict)"("Boolean Text.Text"=w4898) -> ()  [unwired: 2 in, 2 out]
            n3624 = property on="OPEN 2" class="Bool (strict)"("Boolean Text.Text"=w4897) -> ()  [unwired: 2 in, 2 out]
            n3625 = property on="OPEN 3" class="Bool (strict)"("Boolean Text.Text"=w4896) -> ()  [unwired: 2 in, 2 out]
            n3626 = property on="OPEN 4" class="Bool (strict)"("Boolean Text.Text"=w4895) -> ()  [unwired: 2 in, 2 out]
            n3627 = Concatenate Strings(w4880, "\r", w4879) -> ()  [unwired: 1 out]
            n3628 = local read "S 102"() -> (w4853:string)
            n3629 = property on="КОФ1" class="DigNum (strict)"("Caption.Text"=w4893) -> ()  [unwired: 2 in, 2 out]
            n3630 = local read "S 98"() -> (w4857:string)
            n3631 = local read "S 99"() -> (w4856:string)
            n3632 = local read "S 100"() -> (w4855:string)
            n3633 = local read "S 101"() -> (w4854:string)
            n3634 = property on="КОФ2" class="DigNum (strict)"("Caption.Text"=w4892) -> ()  [unwired: 2 in, 2 out]
            n3635 = property on="КОФ3" class="DigNum (strict)"("Caption.Text"=w4891) -> ()  [unwired: 2 in, 2 out]
            n3636 = property on="КОФ4" class="DigNum (strict)"("Caption.Text"=w4890) -> ()  [unwired: 2 in, 2 out]
            n3637 = local read "bs"() -> (w4878:string)
            n3638 = local read "as"() -> (w4877:string)
            n3639 = property on="CH-POWER +" class="DigNum (strict)"("Caption.Text"=w4857) -> ()  [unwired: 2 in, 2 out]
            n3640 = property on="CH-POWER -" class="DigNum (strict)"("Caption.Text"=w4856) -> ()  [unwired: 2 in, 2 out]
            n3641 = property on="CH-HEATER" class="DigNum (strict)"("Caption.Text"=w4855) -> ()  [unwired: 2 in, 2 out]
            n3642 = property on="CH-HUMIDITY DRY" class="DigNum (strict)"("Caption.Text"=w4854) -> ()  [unwired: 2 in, 2 out]
            n3643 = property on="CH-HUMIDITY WET" class="DigNum (strict)"("Caption.Text"=w4853) -> ()  [unwired: 2 in, 2 out]
            n3644 = local read "S 60"() -> (w4889:string)
            n3645 = local read "S 54"() -> (w4899:string)
            n3646 = Concatenate Strings(w4878, "\r", w4877) -> ()  [unwired: 1 out]
            n3647 = Concatenate Strings(w4899, w4889) -> ()  [unwired: 1 out]
            n3648 = local read "S 77"() -> (→"String 43":string)
            n3649 = local read "S 76"() -> (w4872:string)
            n3650 = local read "S 78"() -> (w4871:string)
            n3651 = local read "S 71"() -> (w4883:string)
            n3652 = local read "S 66"() -> (w4888:string)
            n3653 = local read "S 67"() -> (w4887:string)
            n3654 = local read "S 68"() -> (w4886:string)
            n3655 = local read "S 69"() -> (w4885:string)
            n3656 = local read "S 70"() -> (w4884:string)
            n3657 = property on="AIR TEMP" class="DigNum (strict)"("Caption.Text"=w4871) -> ()  [unwired: 2 in, 2 out]
            n3658 = property on="Set Strk" class="DigNum (strict)"("Caption.Text"=w4872) -> ()  [unwired: 2 in, 2 out]
            n3659 = property on="FRIC. FORCE :" class="DigNum (strict)"("Caption.Text"=w4888) -> ()  [unwired: 2 in, 2 out]
            n3660 = property on="TEMPERATURE :" class="DigNum (strict)"("Caption.Text"=w4887) -> ()  [unwired: 2 in, 2 out]
